vi "Srp_Tools_Platform.vi"() -> ()   [LabVIEW 2022 SP3]
panel:
  in  "IPS":refnum<visa-resource-name>
  in  "ITC":refnum<visa-resource-name>
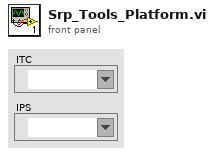
[diagram p1: front panel]
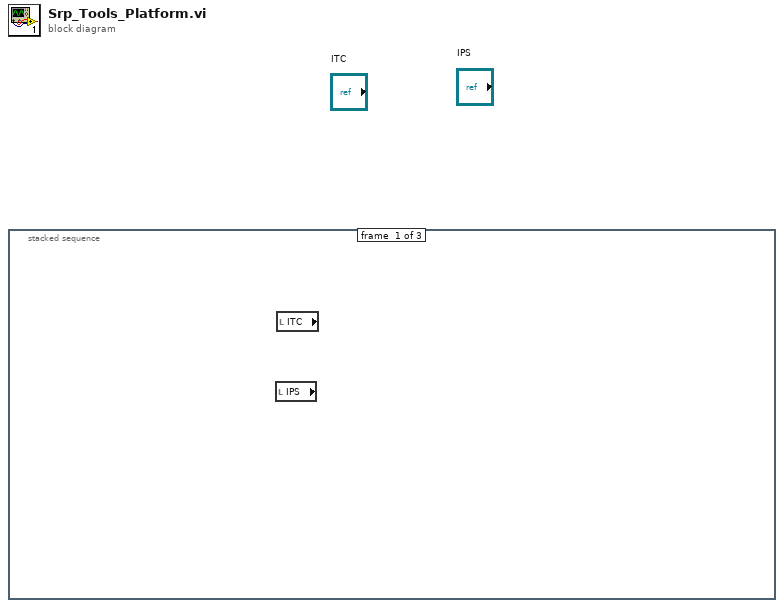
[diagram p0: block diagram]
diagram:
  n1 = stacked-sequence {
    frame #0 {
      n2 = local read "IPS"() -> ()  [unwired: 1 out]
      n3 = local read "ITC"() -> ()  [unwired: 1 out]
    }
    frame #1 {
    }
    frame #2 {
    }
  }
